vi "step7 Solve.vi"(11 "cube in":T1) -> (1 "all corners solved?":bool, 3 "cube out":T1)   [LabVIEW 2011]
uses:
  Typedef/cube.ctl
  Typedef/face.ctl
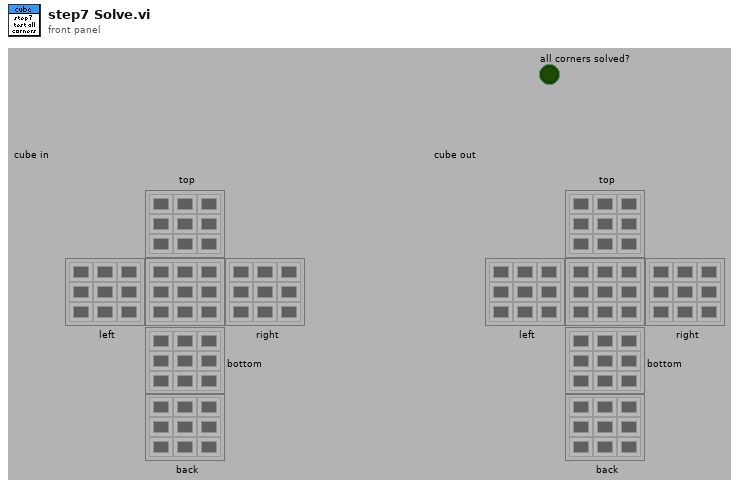
[diagram p1: front panel]
types:
  T1 = typedef "cube.ctl" = cluster{"top":T2, "left":T2, "right":T2, "bottom":T2, "back":T2, "front":T2}
  T2 = typedef "face.ctl" = u32[][]
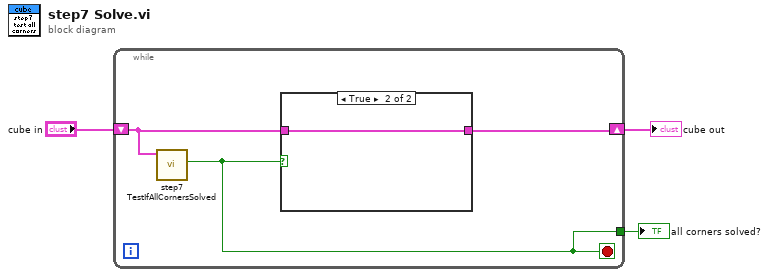
[diagram p0: block diagram]
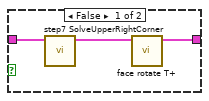
[diagram p2: hidden frame]
diagram:
  n1 = while {
    shift-right: [w5] -> w1
    shift-left: "cube in" -> [w6]
    tunnel: [w4] -> w2
    stop <- w4 stop-if-true
    n2 = call "step7 TestIfAllCornersSolved.vi"("cube in"=w6) -> ("all corners solved?"=w4:bool)  [unwired: 9 in, 1 out]
    n3 = case shown="True" w4 {
      tunnel: [w8 w10] -> w5
      tunnel: w6 -> [w7 w10]
      frame False {
        n4 = call "step7 SolveUpperRightCorner.vi"("cube in"=w7) -> ("cube out"=w9:T1)  [unwired: 10 in]
        n5 = call "face rotate T+.vi"("cube in"=w9) -> ("cube out"=w8:T1)  [unwired: 9 in, 1 out]
      }
      frame True {
      }
    }
  }
  "cube out" <- w1
  "all corners solved?" <- w2
